vi "Create ADS Packet.vi"(4 "Data":u8[](array[numeric]), 5 "State Flag":T2=4 items=["TCP Request"=4, "TCP Response"=5, "UDP Request"=68, "UDP Respone"=69], 6 "Invoke ID":u32, 7 "Command ID":T3=enum."ADS Read Device Info", 8 "Error In":errorcluster, 11 "AMS":T1) -> (0 "Error Out":errorcluster, 3 "ADS Packet":u8[](array[numeric]))   [LabVIEW 2016, in "TwinCAT ADS.lvlib"]
uses:
  TwinCAT ADS.lvlib
  TypeDefs/Command Id.ctl
  TypeDefs/State Flag.ctl
  TypeDefs/AMS.ctl
  TypeDefs/ADS Error.ctl
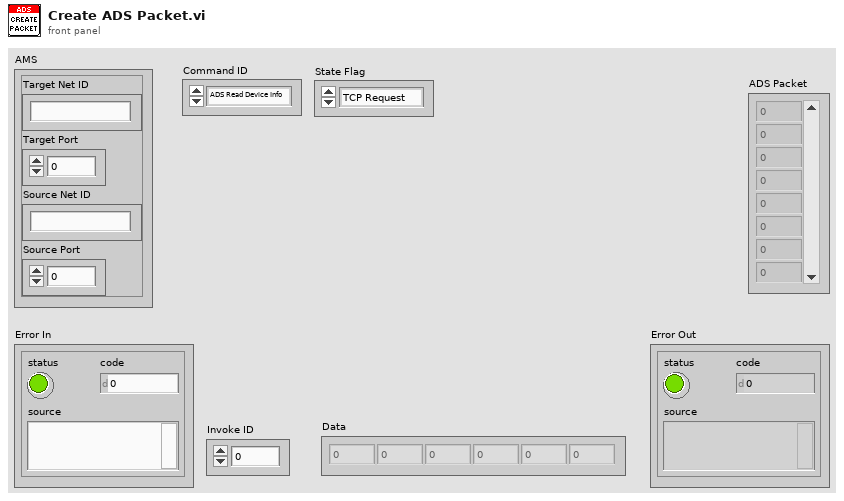
[diagram p1: front panel]
types:
  T1 = typedef "TwinCAT ADS.lvlib/AMS.ctl" = cluster{"Target Net ID":string, "Target Port":u16, "Source Net ID":string, "Source Port":u16}
  T2 = typedef "TwinCAT ADS.lvlib/State Flag.ctl" = u16
  T3 = typedef "TwinCAT ADS.lvlib/Command Id.ctl" = enum16{"Invalid", "ADS Read Device Info", "ADS Read", "ADS Write", "ADS Read State", "ADS Write Control", "ADS Add Device Notification", "ADS Delete Device Notification", "ADS Device Notification", "ADS Read Write"}
  T4 = typedef "TwinCAT ADS.lvlib/ADS Error.ctl" = u32
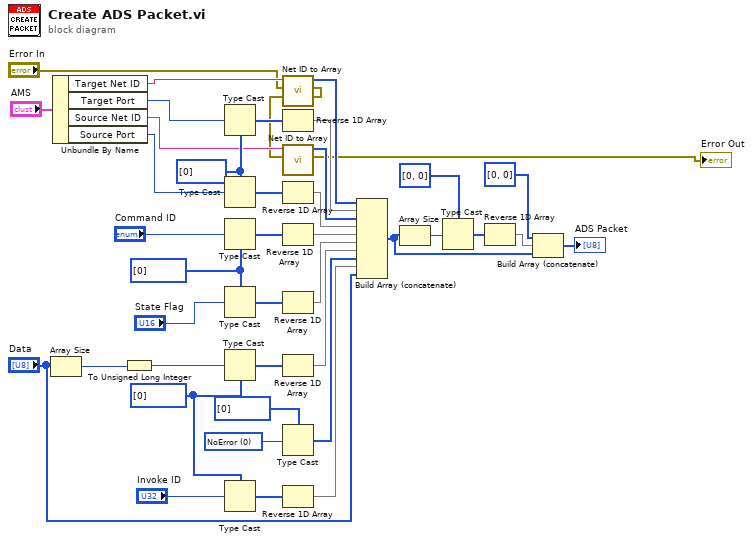
[diagram p0: block diagram]
diagram:
  w1 = T4 0 items=["NoError"=0, "InternalError"=1, "NoRTime"=2, "LockedMemoryError"=3, "MailBoxError"=4, "WrongHMsg"=5, "TargetPortNotFound"=6, "TargetMachineNotFound"=7, "UnknownCommandID"=8, "BadTaskID"=9, "NoIO"=10, "UnknownAmsCommand"=11, "Win32Error"=12, "PortNotConnected"=13, "InvalidAmsLength"=14, "InvalidAmsNetID"=15, "AmsSyncAmsError"=22, "AmsSyncNoIndexMap"=23, "InvalidAmsPort"=24, "NoMemory"=25, "TCPSendError"=26, "HostUnreachable"=27, "NoLockedMemory"=1280, "MailboxFull"=1282, "DeviceError"=1792, "DeviceServiceNotSupported"=1793, "DeviceInvalidGroup"=1794, "DeviceInvalidOffset"=1795, "DeviceInvalidAccess"=1796, "DeviceInvalidSize"=1797, "DeviceInvalidData"=1798, "DeviceNotReady"=1799, "DeviceBusy"=1800, "DeviceInvalidContext"=1801, "DeviceNoMemory"=1802, "DeviceInvalidParam"=1803, "DeviceNotFound"=1804, "DeviceSyntaxError"=1805, "DeviceIncompatible"=1806, "DeviceExists"=1807, "DeviceSymboldNotFound"=1808, "DeviceSymbolVersionInvalid"=1809, "DeviceInvalidState"=1810, "DeviceTransModeNotSupported"=1811, "DeviceNotifyHandleInvalid"=1812, "DeviceClientUnknown"=1813, "DeviceNoMoreHandles"=1814, "DeviceInvalidWatchsize"=1815, "DeviceNotInitialized"=1816, "DeviceTimeOut"=1817, "DeviceNoInterface"=1818, "DeviceInvalidInterface"=1819, "DeviceInvalidCLSID"=1820, "DeviceInvalidObjectID"=1821, "ClientError"=1856, "ClientInvalidParameter"=1857, "ClientListEmpty"=1858, "ClientVariableInUse"=1859, "ClientDuplicateInvokeID"=1860, "ClientSyncTimeOut"=1861, "ClientW32OR"=1862, "ClientTimeoutInvalid"=1863, "ClientPortNotOpen"=1864, "ClientNoAmsAddr"=1865, "ClientSyncInternal"=1872, "ClientAddHash"=1873, "ClientRemoveHash"=1874, "ClientNoMoreSymbols"=1875, "ClientSyncResInvalid"=1876, "ClientSyncPortLocked"=1877, "ClientQueueFull"=1878] ("ADS Error")
  w21 = u8[] [0] ("dimension size")
  w25 = u8[] [0] ("dimension size")
  w39 = u8[] [0] ("dimension size")
  n1 = Array Size(array="Data") -> (size(s)=w30:i32)
  n2 = Unbundle By Name("AMS") -> ("Target Net ID"=w9:string, "Target Port"=w8:u16, "Source Net ID"=w7:string, "Source Port"=w6:u16)
  n3 = To Unsigned Long Integer(number=w30) -> (unsigned 32bit integer=w28:u32)
  n4 = Type Cast(type=w39, x=w8) -> (*(type *) &x=w38:u8[])
  n5 = Type Cast(type=w39, x=w6) -> (*(type *) &x=w37:u8[])
  n6 = Type Cast(type=w25, x="Command ID") -> (*(type *) &x=w33:u8[])
  n7 = Type Cast(type=w25, x="State Flag") -> (*(type *) &x=w31:u8[])
  n8 = Type Cast(type=w21, x=w28) -> (*(type *) &x=w29:u8[])
  n9 = Type Cast(type=w21, x="Invoke ID") -> (*(type *) &x=w23:u8[])
  n10 = call "Net ID to Array.vi"("Error In"="Error In", "Net ID"=w9) -> ("Error Out"=w4:errorcluster, "Net ID (Array)"=w41:u8[])  [unwired: 8 in]
  n11 = Reverse 1D Array(array=w38) -> (reversed array=w36:u8[])
  n12 = call "Net ID to Array.vi"("Error In"=w4, "Net ID"=w7) -> ("Error Out"=→"Error Out":errorcluster, "Net ID (Array)"=w40:u8[])  [unwired: 8 in]
  n13 = Reverse 1D Array(array=w37) -> (reversed array=w35:u8[])
  n14 = Reverse 1D Array(array=w33) -> (reversed array=w27:u8[])
  n15 = Reverse 1D Array(array=w31) -> (reversed array=w26:u8[])
  n16 = Reverse 1D Array(array=w29) -> (reversed array=w24:u8[])
  n17 = Type Cast(type=u8[] [0] ("dimension size"), x=w1) -> (*(type *) &x=w18:u8[])
  n18 = Reverse 1D Array(array=w23) -> (reversed array=w20:u8[])
  n19 = Build Array (concatenate)(w41, w36, w40, w35, w27, w26, w24, w18, w20, "Data") -> (w17:u8[])
  n20 = Array Size(array=w17) -> (size(s)=w11:i32)
  n21 = Type Cast(type=u8[] [0, 0] ("Numeric"), x=w11) -> (*(type *) &x=w15:u8[])
  n22 = Reverse 1D Array(array=w15) -> (reversed array=w13:u8[])
  n23 = Build Array (concatenate)(u8[] [0, 0] ("Numeric"), w13, w17) -> (→"ADS Packet":u8[])
